vi "Tetromino_Create.vi"() -> (15 "Origin":i16, 18 "Tetromino":u8)   [LabVIEW 2018]
uses:
  <vilib>/rvi/Emulation/niFpgaGetClockAttributes.vi
  <vilib>/rvi/Emulation/niFpgaSctlEmulationGetInTimedLoop.vi
  <vilib>/rvi/Emulation/niFpgaEmulationReportErrorSimple.vi
  <vilib>/rvi/Emulation/niFpgaCriticalErrorInLSC.vi
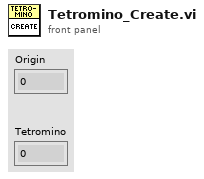
[diagram p1: front panel]
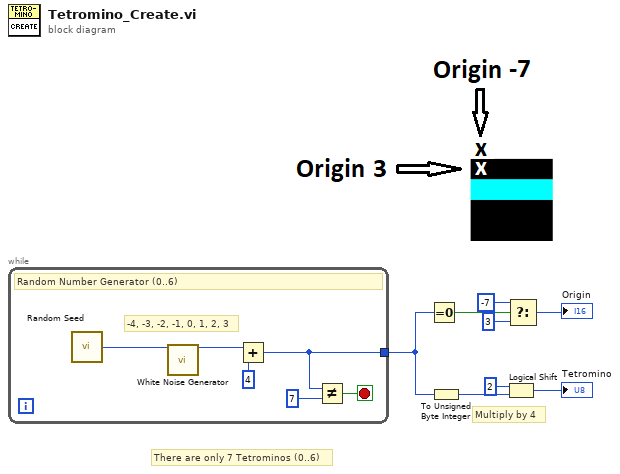
[diagram p0: block diagram]
diagram:
  # "There are only 7 Tetrominos (0..6)"
  # "Multiply by 4"
  n1 = while {
    tunnel: [w10] -> w4
    stop <- w13 stop-if-true
    # "-4, -3, -2, -1, 0, 1, 2, 3"
    # "Random Number Generator (0..6)"
    n2 = call "Random Seed"() -> ("Tick Count(Ticks)"=w9:u32)
    n3 = call "White Noise Generator"("seed"=w9) -> ("white noise out"=w11:i16)  [unwired: 14 in]
    n4 = Add(x=w11, y=i16 4) -> (x+y=w10:i16)
    n5 = Not Equal?(x=w10, y=i16 7) -> (x != y?=w13:bool)
  }
  n6 = Equal To 0?(x=w4) -> (x = 0?=w6:bool)
  n7 = To Unsigned Byte Integer(number=w4) -> (unsigned 8bit integer=w3:u8)
  n8 = Logical Shift(y=i16 2, x=w3) -> (x << y=→"Tetromino":u8)
  n9 = Select(t=i16 -7, s=w6, f=i16 3 ("Origin")) -> (s? t:f=→"Origin":i16)
